vi "LV to ITX  Graph.vi"(4 "Trace Names (XY Graph Only)":string[](array[string])=["first", "second", "third"], 6 "X,Y,Z Scale Names":string[](array[string])=["X", "Y", "Z"], 7 "Enum":enum16{"XY Graph", "Intensity Graph"}(ring), 8 "Intensity Graph":dbl[][](graph), 9 "XY Graph":cluster{dbl[], dbl[]}[](graph), 10 "Filename":string="testname", 11 "Path":path=path "C:/temp") -> ()   [LabVIEW 2016, in "LVtoITX.lvclass"]
uses:
  LVtoITX.lvclass
panel:
  out "Tab":enum32{"XY Graph", "Intensity Graph"}(tab)
  in  "open file in Igor?":bool
  # "<-- choose which graph you would like to save"
  # "Igor Syntax:\n\\S = superscript\n\\B = subscript\n\\M = normal\n\nExample:\nV\\MS\\B = \"V_S\""
  # "adjust offset and multiplier\nhere to make your graph look\ncorrect in Igor"
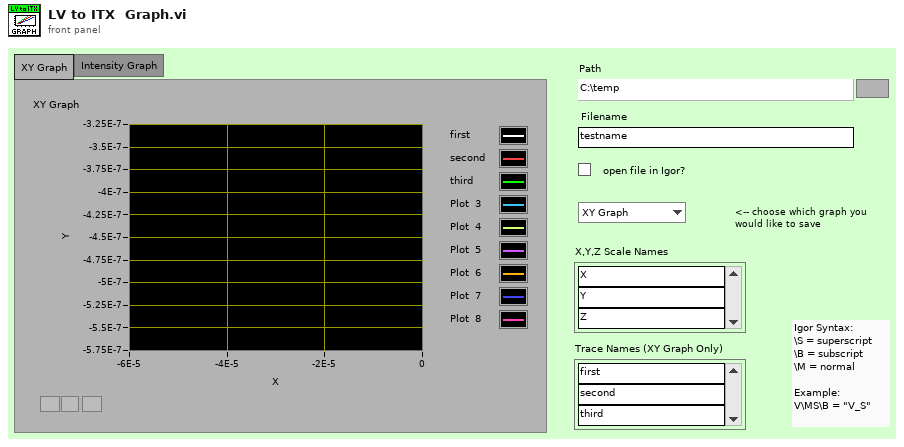
[diagram p1: front panel]
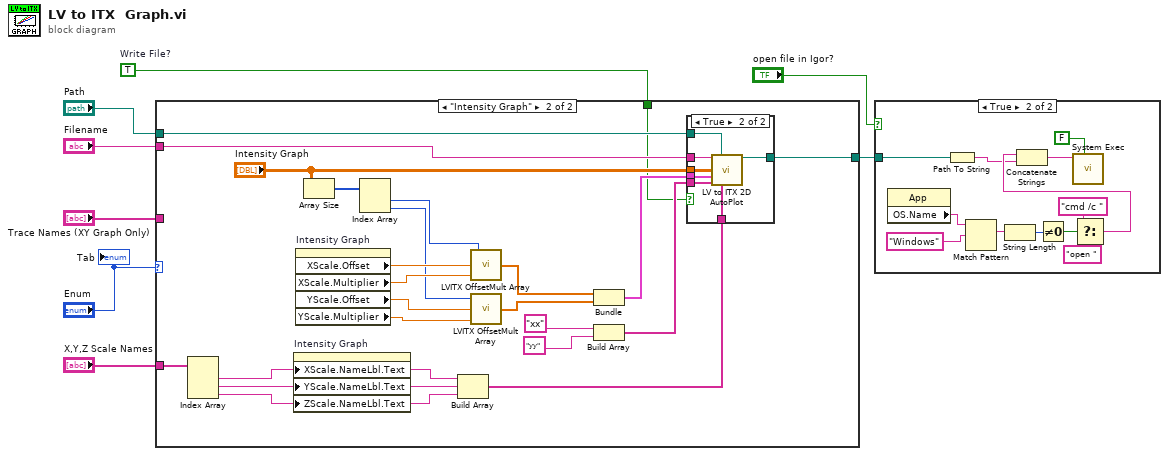
[diagram p0: block diagram]
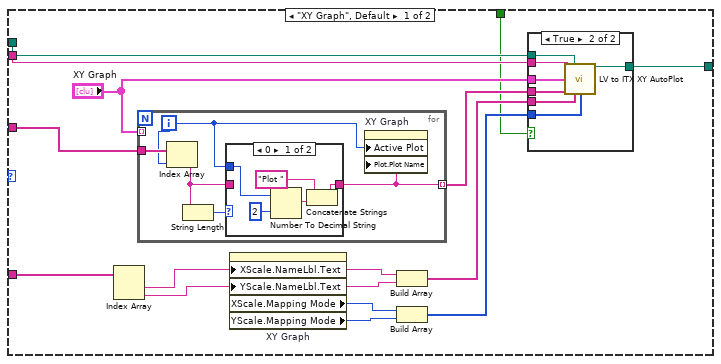
[diagram p3: hidden frame]
diagram:
  w3 = TRUE  # Write File?
  n1 = case shown="\"Intensity Graph\"" "Enum" {
    tunnel: "Path" -> [w22 w47]
    tunnel: "Filename" -> [w21 w64]
    tunnel: [w19 w54] -> w7
    tunnel: "X,Y,Z Scale Names" -> [w13 w46]
    tunnel: w3 -> [w10 w42]
    tunnel: "Trace Names (XY Graph Only)" -> [w9 _]
    frame "XY Graph", Default {
      n2 = Index Array(array=w13) -> (element #1=w12:string, element #2=w11:string)  [unwired: 2 in]
      n3 = for {
        tunnel: "XY Graph" -> [_] mode=indexing
        tunnel: [w33] -> w18 mode=indexing
        tunnel: w9 -> [w35]
        i -> [w31]
        n4 = Index Array(array=w35, index=w31) -> (element=w32:string)
        n5 = String Length(string=w32) -> (length=w34:i32)
        n6 = case shown="0" w34 {
          tunnel: [w38 w41] -> w33
          tunnel: w32 -> [_ w41]
          tunnel: w31 -> [w36 _]
          frame 0 {
            n7 = Number To Decimal String(number=w36, width (-)=i16 2) -> (decimal integer string=w39:string)
            n8 = Concatenate Strings("Plot " ("decimal integer string"), w39) -> (w38:string)
          }
          frame 1, Default {
          }
        }
        n9 = property on="XY Graph" class="XYGraph (strict)"("Active Plot"=w31, "Plot.Plot Name"=w33) -> ()  [unwired: 2 in, 2 out]
      }
      n10 = property on="XY Graph" class="XYGraph (strict)"("XScale.NameLbl.Text"=w12, "YScale.NameLbl.Text"=w11) -> ("XScale.Mapping Mode"=w16:u8, "YScale.Mapping Mode"=w15:u8)  [unwired: 2 in, 2 out]
      n11 = Build Array(w12, w11) -> (w17:string[])
      n12 = Build Array(w16, w15) -> (w14:u8[])
      n13 = case shown="True" w10 {
        tunnel: w22 -> [w23 w30]
        tunnel: w21 -> [_ w29]
        tunnel: "XY Graph" -> [_ w28]
        tunnel: [w23 w27] -> w19
        tunnel: w18 -> [_ w26]
        tunnel: w17 -> [_ w25]
        tunnel: w14 -> [_ w24]
        frame False {
        }
        frame True {
          n14 = call "LV to ITX XY AutoPlot.vi"("filename"=w29, "path"=w30, "XY Array"=w28, "wavenames (.Vx, etc)"=w26, "X,Y Labels"=w25, "X,Y Log"=w24) -> ("file"=w27:path)  [unwired: 9 in]
        }
      }
    }
    frame "Intensity Graph" {
      n15 = Index Array(array=w46) -> (element #1=w44:string, element #2=w45:string, element #3=w43:string)  [unwired: 3 in]
      n16 = property on="Intensity Graph" class="IntGraph (strict)"("XScale.NameLbl.Text"=w44, "YScale.NameLbl.Text"=w45, "ZScale.NameLbl.Text"=w43) -> ()  [unwired: 2 in, 2 out]
      n17 = property on="Intensity Graph" class="IntGraph (strict)"() -> ("XScale.Offset"=w60:dbl, "XScale.Multiplier"=w59:dbl, "YScale.Offset"=w57:dbl, "YScale.Multiplier"=w56:dbl)  [unwired: 2 in, 2 out]
      n18 = Array Size(array="Intensity Graph") -> (size(s)=w61:i32[])
      n19 = Index Array(array=w61) -> (element #1=w58:i32, element #2=w48:i32)  [unwired: 2 in]
      n20 = Build Array(w44, w45, w43) -> (w63:string[])
      n21 = call "LVITX OffsetMult Array.vi"("XScale.Multiplier"=w59, "XScale.Offset"=w60, "Array Size"=w58) -> ("Array"=w52:dbl[])
      n22 = call "LVITX OffsetMult Array.vi"("XScale.Multiplier"=w56, "XScale.Offset"=w57, "Array Size"=w48) -> ("Array"=w53:dbl[])
      n23 = Bundle("Array"=w52, "Array"=w53) -> (w55:cluster{"Array":dbl[], "Array":dbl[]})  [unwired: 1 in]
      n24 = Build Array("xx" ("X Scale.Name Label.Text"), "yy" ("X Scale.Name Label.Text")) -> (w51:string[])
      n25 = case shown="True" w42 {
        tunnel: w64 -> [_ w72]
        tunnel: w63 -> [_ w71]
        tunnel: "Intensity Graph" -> [_ w70]
        tunnel: w55 -> [_ w69]
        tunnel: [w65 w68] -> w54
        tunnel: w51 -> [_ w67]
        tunnel: w47 -> [w65 w66]
        frame False {
        }
        frame True {
          n26 = call "LV to ITX 2D AutoPlot.vi"("filename"=w72, "path"=w66, "2D Array"=w70, "X, Y Arrays"=w69, "X, Y wavenames"=w67, "X,Y,Z Labels"=w71) -> ("file"=w68:path)  [unwired: 9 in]
        }
      }
    }
  }
  n27 = case shown="True" "open file in Igor?" {
    tunnel: w7 -> [_ w76]
    frame False {
    }
    frame True {
      n28 = property class="App"() -> ("OS.Name"=w77:string)  [unwired: 2 in, 2 out]
      n29 = Path To String(path=w76) -> (string=w73:string)
      n30 = Match Pattern(string=w77, regular expression="Windows") -> (match substring=w83:string)  [unwired: 1 in, 3 out]
      n31 = String Length(string=w83) -> (length=w82:i32)
      n32 = Not Equal To 0?(x=w82) -> (x != 0?=w80:bool)
      n33 = Select(t="cmd /c ", s=w80, f="open ") -> (s? t:f=w75:string)
      n34 = Concatenate Strings(w75, w73) -> (w84:string)
      n35 = call <vilib>:"System Exec.vi"("wait until completion? (T)"=FALSE, "command line"=w84) -> ()  [unwired: 6 in, 4 out]
    }
  }
  "Tab" <- "Enum"
